vi "Check VI Error.vi"(8 "error in (no error)":errorcluster, 11 "VI Ref":refnum<vi>) -> (0 "error out":errorcluster)   [LabVIEW 2025, in "I2C Bus Monitor UI.lvlib"]
uses:
  I2C Bus Monitor UI.lvlib
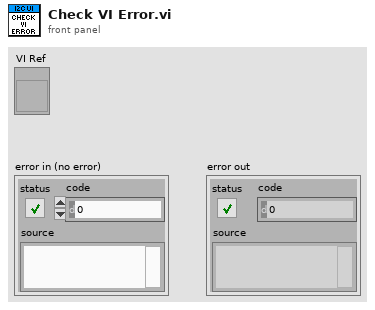
[diagram p1: front panel]
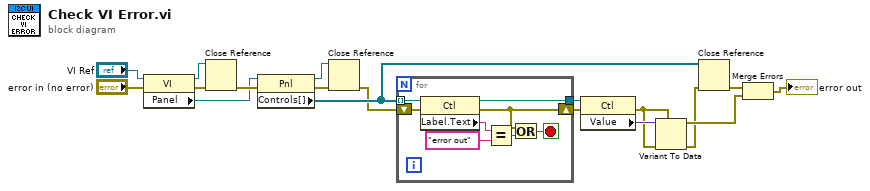
[diagram p0: block diagram]
diagram:
  n1 = property class="VI"(reference="VI Ref", error in="error in (no error)") -> (reference out=w9:refnum<vi>, error out=w4:errorcluster, "Panel"=w3:refnum<vi>)
  n2 = Close Reference(reference=w9, error in (no error)=w4) -> (error out=w8:errorcluster)
  n3 = property class="Pnl"(reference=w3, error in=w8) -> (reference out=w11:refnum<vi>, error out=w5:errorcluster, "Controls[]"=w13:refnum<vi>[])
  n4 = Close Reference(reference=w11, error in (no error)=w5) -> (error out=w10:errorcluster)
  n5 = for {
    tunnel: w13 -> [w26] mode=indexing
    tunnel: [w23] -> w7
    shift-right: [w19] -> w6
    shift-left: w10 -> [w21]
    stop <- w20 stop-if-true
    n6 = property class="Ctl"(reference=w26, error in=w21) -> (reference out=w23:refnum<vi>, error out=w19:errorcluster, "Label.Text"=w25:string)
    n7 = Equal?(x=w25, y="error out" ("Label.Text")) -> (x = y?=w22:bool)
    n8 = Or(x=w19, y=w22) -> (x .or. y?=w20:bool)
  }
  n9 = property class="Ctl"(reference=w7, error in=w6) -> (error out=w17:errorcluster, "Value"=w18:variant)  [unwired: 1 out]
  n10 = Variant To Data(error in=w17, type=w17, Variant=w18) -> (data=w16:errorcluster, error out=w15:errorcluster)
  n11 = Close Reference(reference=w13, error in (no error)=w15) -> (error out=w12:errorcluster)
  n12 = Merge Errors(w12, w16) -> (→"error out":errorcluster)
